vi "UnnameTypeDescriptor.vi"(2 "error in (no error)":errorcluster, 3 "type string":i16[](array[numeric])) -> (0 "error out":errorcluster, 1 "unnamed type string":i16[](array[numeric]))   [LabVIEW 2017]
doc: "Removes a data name from the type descriptor. Not all types have been implemented, only those for which LVHDF5 writes the type descriptor into the file."
panel:
  # "LVHDF5 Toolkit\nCopyright (c) 2005-2013 by Jason D. Sommerville\nCopyright (c) 2014 by UPVI, LLC.\n\nThis use and distribution of this file is governed by the terms found in \nLICENSE.txt distributed with this toolkit and installed at\n <user.lib>\\_lvhdf5\\LICENSE.txt"
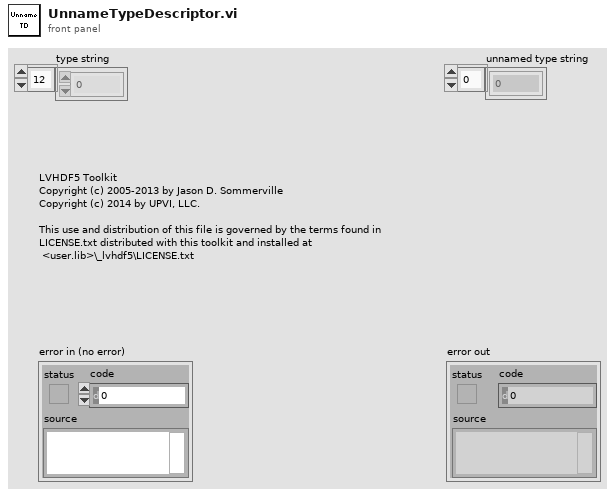
[diagram p1: front panel]
types:
  T1 = enum16{"<Null>", "I8", "I16", "I32", "I64", "U8", "U16", "U32", "U64", "SGL", "DBL", "EXT", "CSG", "CDB", "CXT", "0x0F", "0x10", "0x11", "0x12", "0x13", "0x14", "Enum U8", "Enum U16", "Enum U32", "Enum U64", "SGL PQ", "DBL PQ", "EXT PQ", "CSG PQ", "CDB PQ", "CXT PQ", "0x1F", "0x20", "Boolean", "0x22", "0x23", "0x24", "0x25", "0x26", "0x27", "0x28", "0x29", "0x2A", "0x2B", "0x2C", "0x2D", "0x2E", "0x2F", "String", "0x31", "Path", "Pict", "0x34", "0x35", "0x36", "DAQ", "0x38", "0x39", "0x3A", "0x3B", "0x3C", "0x3D", "0x3E", "0x3F", "Array", "0x41", "0x42", "0x43", "0x44", "0x45", "0x46", "0x47", "0x48", "0x49", "0x4A", "0x4B", "0x4C", "0x4D", "0x4E", "0x4F", "Cluster", "0x51", "0x52", "Variant", "Waveform", "0x55", "0x56", "0x57", "0x58", "0x59", "0x5A", "0x5B", "0x5C", "0x5D", "0x5E", "0x5F", "0x60", "0x61", "0x62", "0x63", "0x64", "0x65", "0x66", "0x67", "0x68", "0x69", "0x6A", "0x6B", "0x6C", "0x6D", "0x6E", "0x6F", "Refnum"}
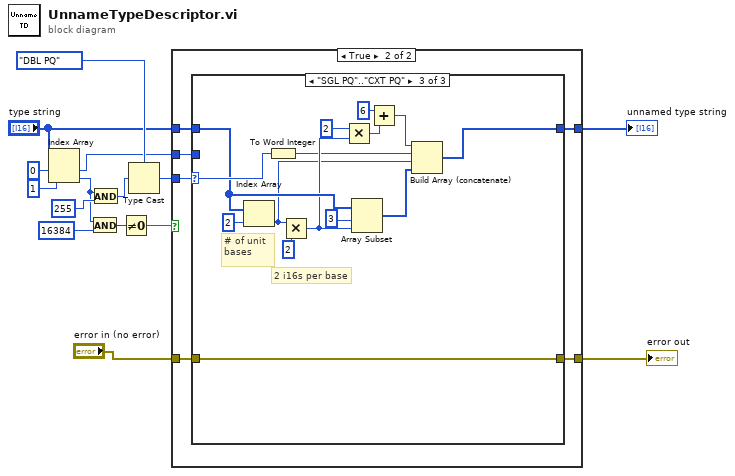
[diagram p0: block diagram]
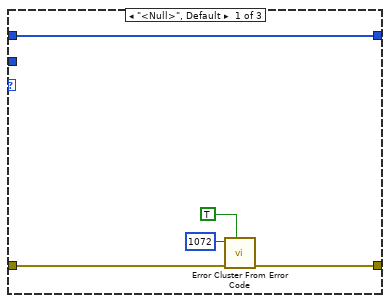
[diagram p3: hidden frame]
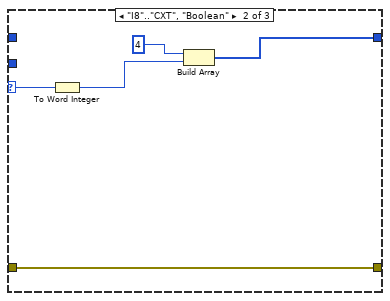
[diagram p4: hidden frame]
diagram:
  n1 = Index Array(array="type string", index #1=0 ("index"), index #2=1 ("index")) -> (element #1=w2:i16, element #2=w8:i16)
  n2 = And(x=w8, y=i16 16384) -> (x .and. y?=w6:i16)
  n3 = And(x=w8, y=i16 255) -> (x .and. y?=w1:i16)
  n4 = Not Equal To 0?(x=w6) -> (x != 0?=w5:bool)
  n5 = Type Cast(type=T1."DBL PQ" ("Type Descriptor Enumeration"), x=w1) -> (*(type *) &x=w12:T1)
  n6 = case shown="True" w5 {
    tunnel: w12 -> [_ w23]
    tunnel: "error in (no error)" -> [w17 w22]
    tunnel: [w17 w21] -> w10
    tunnel: [w16 w18] -> w4
    tunnel: "type string" -> [w16 w20]
    tunnel: w2 -> [_ w19]
    frame False {
    }
    frame True {
      n7 = case shown="\"SGL PQ\"..\"CXT PQ\"" w23 {
        selector: w23 -> [_ w31 w47]
        tunnel: w22 -> [w26 w33 w48]
        tunnel: [w25 w33 w48] -> w21
        tunnel: w20 -> [w24 _ w43]
        tunnel: w19 -> [_ _ _]
        tunnel: [w24 w30 w46] -> w18
        frame "<Null>", Default {
          n8 = call <vilib>:"Error Cluster From Error Code.vi"("show call chain? (False)"=TRUE, "error in (no error)"=w26, "error code (0)"=1072) -> ("error out"=w25:errorcluster)  [unwired: 6 in]
        }
        frame "I8".."CXT", "Boolean" {
          n9 = To Word Integer(number=w31) -> (16bit integer=w29:i16)
          n10 = Build Array(i16 4, w29) -> (w30:i16[])
        }
        frame "SGL PQ".."CXT PQ" {
          # "2 i16s per base"
          # "# of unit bases"
          n11 = Index Array(array=w43, index=2) -> (element=w36:i16)
          n12 = To Word Integer(number=w47) -> (16bit integer=w34:i16)
          n13 = Multiply(x=w36, y=i16 2) -> (x*y=w40:i16)
          n14 = Multiply(x=i16 2, y=w40) -> (x*y=w38:i16)
          n15 = Array Subset(array=w43, index=3, length=w40) -> (w35:i16[])
          n16 = Add(x=i16 6, y=w38) -> (x+y=w37:i16)
          n17 = Build Array (concatenate)(w37, w34, w36, w35) -> (w46:i16[])
        }
      }
    }
  }
  "unnamed type string" <- w4
  "error out" <- w10
